vi "Setup Statically-Linked subWorkers.vi"(8 "error in":errorcluster, 11 "TCP Server Example in":refnum<class "TCP Server Example.lvclass">) -> (0 "error out":errorcluster, 3 "TCP Server Example out":refnum<class "TCP Server Example.lvclass">)   [LabVIEW 2017, in "TCP Server Example.lvclass"]
doc: "This VI performs a setup of all the statically-linked subWorkers that belong to the Worker that owns this VI. This VI must be called <b>before</b> any statically-linked subWorkers are called."
uses:
  TCP Server Example.lvclass
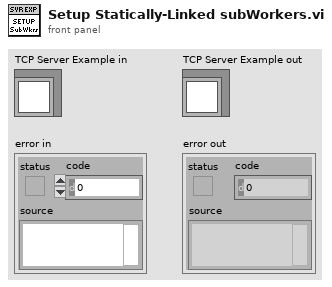
[diagram p1: front panel]
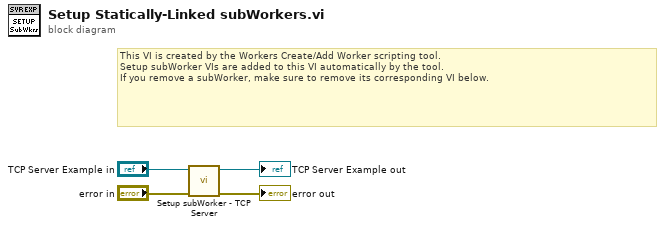
[diagram p0: block diagram]
diagram:
  # "This VI is created by the Workers Create/Add Worker scripting tool.\nSetup subWorker VIs are added to this VI automatically by the tool.\nIf you remove a subWorker, make sure to remove its corresponding VI below."
  n1 = call "Setup subWorker - TCP Server.vi"("error in"="error in", "TCP Server Example in"="TCP Server Example in") -> ("error out"=→"error out":errorcluster, "TCP Server Example out"=→"TCP Server Example out":refnum<class "TCP Server Example.lvclass">)  [unwired: 8 in]
